vi "Init FPGATarget.vi"(6 "instVIref":T1, 9 "target structure name":string, 11 "FPGAtarget in":refnum<class "FPGATarget.lvclass">) -> (3 "FPGAtarget out":refnum<class "FPGATarget.lvclass">)   [LabVIEW 2020, in "NI_TargetHelper.lvlib" / "FPGATarget.lvclass"]
uses:
  <vilib>/TargetSupport/NI_TargetHelper/FPGATarget/FPGATarget.lvclass
  <vilib>/TargetSupport/NI_TargetHelper/Instance VIref.ctl
  <vilib>/TargetSupport/NI_TargetHelper/FPGATarget/FPGATarget.lvclass/FPGATarget.ctl
  <vilib>/TargetSupport/NI_TargetHelper/NI_TargetHelper.lvlib
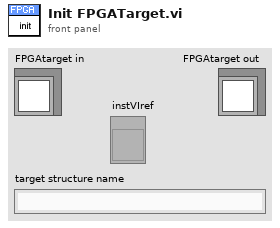
[diagram p1: front panel]
types:
  T1 = typedef "NI_TargetHelper.lvlib/Instance VIref.ctl" = refnum<vi>
  T2 = enum32{"invalid VI type", "Standard VI", "Control VI", "Global VI", "Polymorphic VI", "Configuration VI", "SubSystem", "Facade VI", "Method VI", "Statechart Diagram VI"}
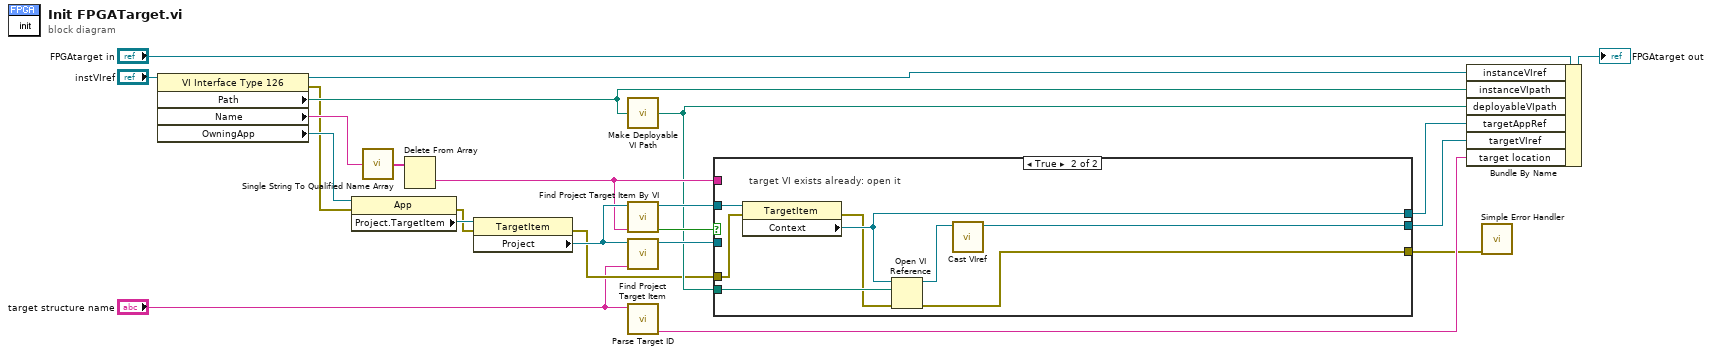
[diagram p0: block diagram]
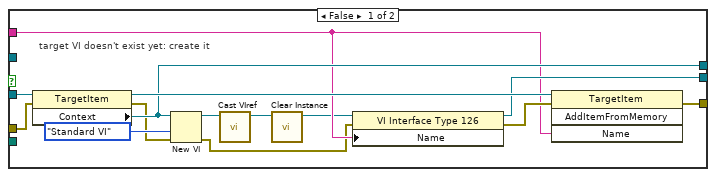
[diagram p2: hidden frame]
diagram:
  n1 = property class="VI Interface Type 126"(reference="instVIref") -> (reference out=w18:T1, error out=w8:errorcluster, "Path"=w16:path, "Name"=w21:string, "OwningApp"=w20:refnum<vi>)  [unwired: 1 in]
  n2 = property class="App"(reference=w20, error in=w8) -> (error out=w7:errorcluster, "Project.TargetItem"=w22:refnum<vi>)  [unwired: 1 out]
  n3 = call <vilib>:"Single String To Qualified Name Array.vi"("Fully Qualified String"=w21) -> ("Fully Qualified Array"=w23:string[])
  n4 = Delete From Array(array=w23) -> (deleted portion=w11:string)  [unwired: 2 in, 1 out]
  n5 = property class="TargetItem"(reference=w22, error in=w7) -> (error out=w6:errorcluster, "Project"=w15:refnum<vi>)  [unwired: 1 out]
  n6 = call <vilib>:"Make Deployable VI Path.vi"("instance path"=w16) -> ("deployable path"=w9:path)
  n7 = call <vilib>:"Find Project Target Item By VI.vi"("vi name"=w11, "project"=w15) -> ("found"=w14:bool, "TargetItem Refnum"=w10:refnum<vi>)  [unwired: 8 in]
  n8 = call <vilib>:"Find Project Target Item.vi"("target structure name"="target structure name", "project"=w15) -> ("TargetItem Refnum"=w19:refnum<vi>)  [unwired: 8 in, 1 out]
  n9 = call <vilib>:"Parse Target ID.vi"("targetID"="target structure name") -> ("target location"=w17:string)  [unwired: 9 in, 1 out]
  n10 = case shown="True" w14 {
    tunnel: w19 -> [w37 _]
    tunnel: w11 -> [w31 _]
    tunnel: [w33 w38] -> w13
    tunnel: [w32 w44] -> w12
    tunnel: w10 -> [_ w45]
    tunnel: w9 -> [_ w43]
    tunnel: w6 -> [w29 w42]
    tunnel: [w24 w40] -> w5
    frame False {
      # "target VI doesn't exist yet: create it"
      n11 = property class="TargetItem"(reference=w37, error in=w29) -> (reference out=w35:refnum<vi>, error out=w28:errorcluster, "Context"=w32:refnum<vi>)
      n12 = New VI(8:w28, 9:T2."Standard VI" ("vi type (standard vi)"), 11:w32) -> (0:w27:errorcluster, 3:w30:refnum<vi>)  [unwired: 4 in]
      n13 = call <vilib>:"Cast VIref.vi"("VI Refnum"=w30) -> ("instVIref"=w26:T1)  [unwired: 10 in]
      n14 = call <vilib>:"Clear Instance.vi"("instVIref"=w26) -> ("instVIref out"=w25:T1)  [unwired: 9 in, 1 out]
      n15 = property class="VI Interface Type 126"(reference=w25, error in=w27, "Name"=w31) -> (reference out=w33:T1, error out=w34:errorcluster)
      n16 = invoke class="TargetItem" method="AddItemFromMemory"(reference=w35, error in=w34, "Name"=w31) -> (error out=w24:errorcluster)  [unwired: 1 in, 3 out]
    }
    frame True {
      # "target VI exists already: open it"
      n17 = property class="TargetItem"(reference=w45, error in=w42) -> (error out=w41:errorcluster, "Context"=w44:refnum<vi>)  [unwired: 1 out]
      n18 = Open VI Reference(application reference (local)=w44, vi path=w43, error in (no error)=w41) -> (vi reference=w39:refnum<vi>, error out=w40:errorcluster)  [unwired: 3 in]
      n19 = call <vilib>:"Cast VIref.vi"("VI Refnum"=w39) -> ("instVIref"=w38:T1)  [unwired: 10 in]
    }
  }
  n20 = Bundle By Name(cluster="FPGAtarget in", "instanceVIref"=w18, "instanceVIpath"=w16, "deployableVIpath"=w9, "targetAppRef"=w12, "targetVIref"=w13, "target location"=w17) -> (→"FPGAtarget out":refnum<class "FPGATarget.lvclass">)
  n21 = call <vilib>:"Simple Error Handler.vi"("error in (no error)"=w5) -> ()  [unwired: 4 in, 5 out]
